vi "写入经历时间.vi"(8 "error in (no error)":errorcluster caption="错误输入（无错误）", 10 "经历时间":dbl, 11 "定时器类输入":refnum<class "定时器类.lvclass">) -> (0 "error out":errorcluster caption="错误输出", 3 "定时器类输出":refnum<class "定时器类.lvclass">)   [LabVIEW 2014]
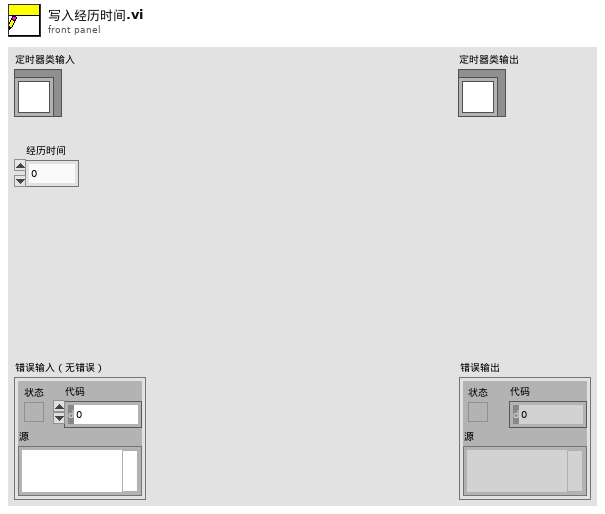
[diagram p1: front panel]
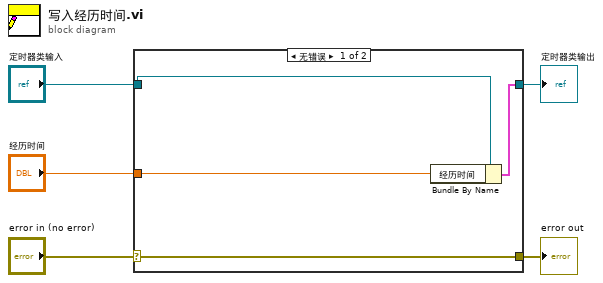
[diagram p0: block diagram]
diagram:
  n1 = case shown="无错误" "error in (no error)" {
    selector: "error in (no error)" -> [w9 w10]
    tunnel: [w9 w10] -> w4
    tunnel: [w7 w11] -> w2
    tunnel: "定时器类输入" -> [w8 w11]
    tunnel: "经历时间" -> [w6 _]
    frame No Error {
      n2 = Bundle By Name(cluster=w8, "经历时间"=w6) -> (w7:cluster{})
    }
    frame Error {
    }
  }
  "error out" <- w4
  "定时器类输出" <- w2
